vi "Get sr850 Formated Parameters.VI"(8 "error in (no error)":errorcluster, 10 "Initial String":string, 11 "VISA Resource Name":refnum<visa-resource-name>) -> (0 "error out":errorcluster, 1 "Time Constant":dbl format="%.2e", 2 "Sensitivity":dbl format="%.4e", 3 "Frequency":dbl format="%.2e", 4 "Phase":dbl format="%.2f", 5 "Oscillator voltage":dbl format="%.2e", 6 "Parameters":string="SR850 Lockin Settings", 7 "Filter Slope":i32, 9 "Data titles":string[](array[string])=["SRS_Vx (V)", "SRS_Vy (V)"])   [LabVIEW 2015]
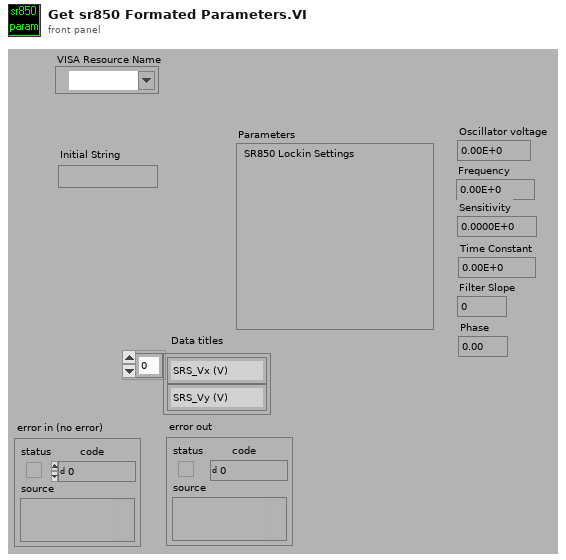
[diagram p1: front panel]
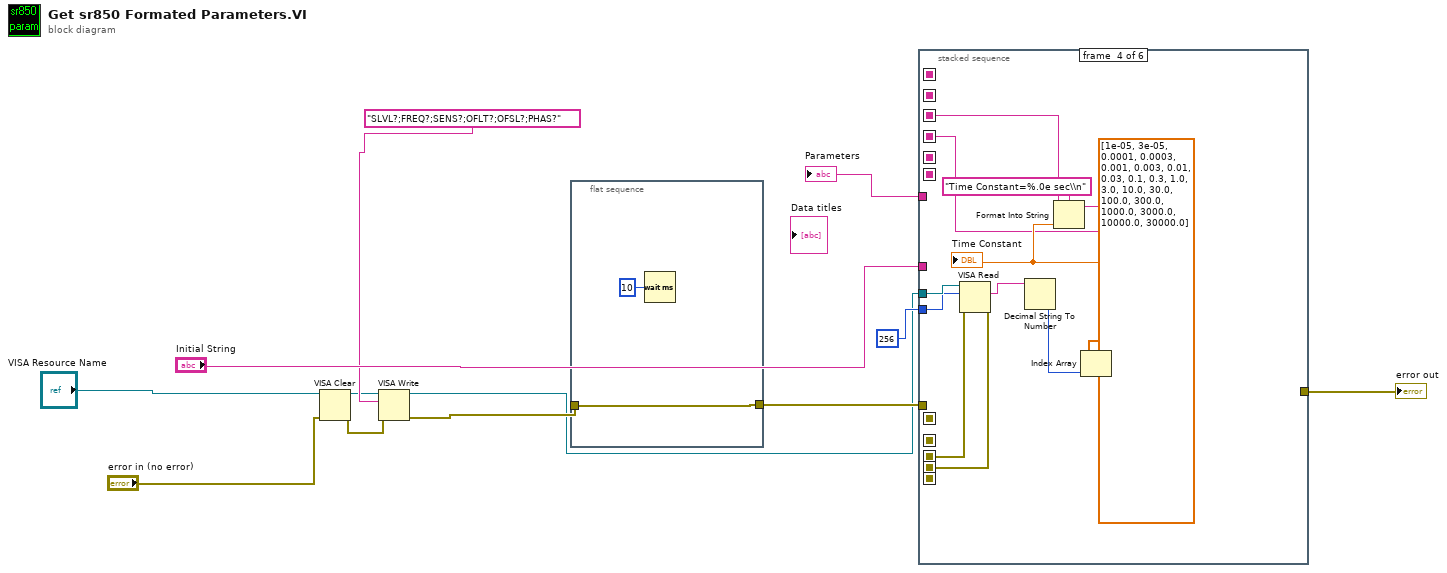
[diagram p0: block diagram]
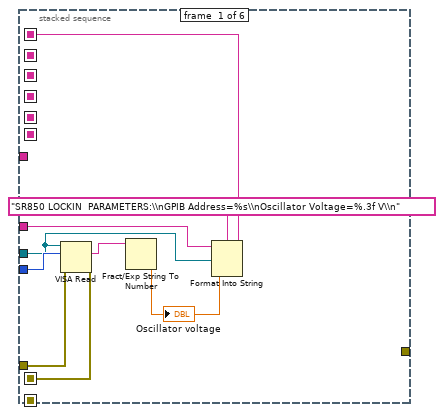
[diagram p2: hidden frame]
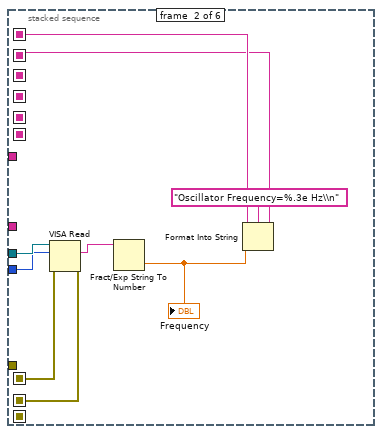
[diagram p3: hidden frame]
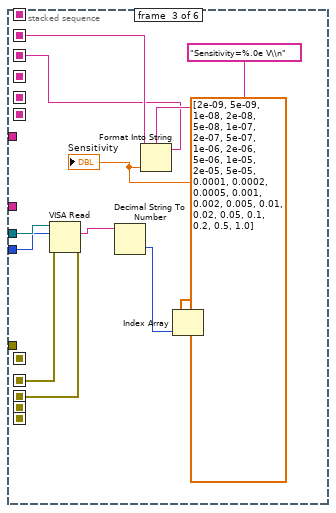
[diagram p4: hidden frame]
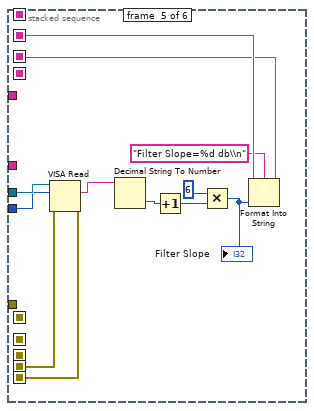
[diagram p5: hidden frame]
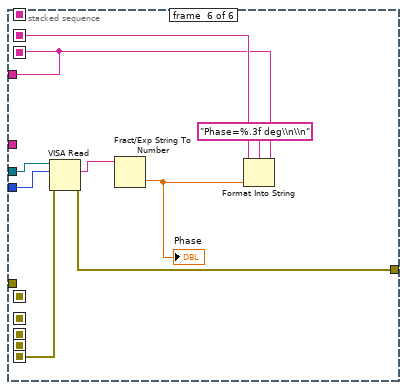
[diagram p6: hidden frame]
diagram:
  n1 = VISA Clear(VISA resource name="VISA Resource Name", error in (no error)="error in (no error)") -> (VISA resource name out=w3:refnum<visa-resource-name>, error out=w6:errorcluster)
  n2 = VISA Write(VISA resource name=w3, write buffer="SLVL?;FREQ?;SENS?;OFLT?;OFSL?;PHAS?" ("data string"), error in (no error)=w6) -> (VISA resource name out=w1:refnum<visa-resource-name>, error out=w5:errorcluster)  [unwired: 1 out]
  n3 = flat-sequence {
    tunnel: [w13] -> w7
    tunnel: w5 -> [w13]
    frame #0 {
      n4 = Wait (ms)(milliseconds to wait=u32 10) -> ()  [unwired: 1 out]
    }
  }
  n5 = stacked-sequence {
    seq-local: [w21 _ _ _ _ _] -> [_ w29 _ _ _ _]
    seq-local: [_ w28 _ _ _ _] -> [_ _ w37 _ _ _]
    seq-local: [_ _ w36 _ _ _] -> [_ _ _ w48 _ _]
    seq-local: [_ _ _ w47 _ _] -> [_ _ _ _ w60 _]
    seq-local: [_ _ _ _ w59 _] -> [_ _ _ _ _ w72]
    seq-local: [_ _ _ _ _ w71] -> [_ _ _ _ _ _]
    seq-local: [w18 _ _ _ _ _] -> [_ w26 _ _ _ _]
    seq-local: [_ w25 _ _ _ _] -> [_ _ w35 _ _ _]
    seq-local: [_ _ w34 _ _ _] -> [_ _ _ w46 _ _]
    seq-local: [_ _ _ w45 _ _] -> [_ _ _ _ w57 _]
    seq-local: [_ _ _ _ w56 _] -> [_ _ _ _ _ w70]
    tunnel: w1 -> [w16 w32 w43 w54 w66 w68]
    tunnel: u32 256 ("count") -> [w23 w27 w42 w53 w65 w75]
    tunnel: [_ _ _ _ _ w71] -> w8
    tunnel: "Initial String" -> [w20 _ _ _ _ _]
    tunnel: w7 -> [w19 _ _ _ _ _]
    tunnel: [_ _ _ _ _ w69] -> w9
    frame #0 {
      n6 = VISA Read(VISA resource name=w16, byte count=w23, error in (no error)=w19) -> (read buffer=w15:string, error out=w18:errorcluster)  [unwired: 2 out]
      n7 = Fract/Exp String To Number(string=w15) -> (number=w17:dbl)  [unwired: 4 out]
      "Oscillator voltage" <- w17
      n8 = Format Into String(format string="SR850 LOCKIN  PARAMETERS:\\nGPIB Address=%s\\nOscillator Voltage=%.3f V\\n", initial string=w20, w16, w17) -> (resulting string=w21:string)  [unwired: 1 in, 1 out]
    }
    frame #1 {
      n9 = VISA Read(VISA resource name=w32, byte count=w27, error in (no error)=w26) -> (read buffer=w24:string, error out=w25:errorcluster)  [unwired: 2 out]
      n10 = Fract/Exp String To Number(string=w24) -> (number=w30:dbl)  [unwired: 4 out]
      "Frequency" <- w30
      n11 = Format Into String(format string="Oscillator Frequency=%.3e Hz\\n", initial string=w29, w30) -> (resulting string=w28:string)  [unwired: 1 in, 1 out]
    }
    frame #2 {
      n12 = VISA Read(VISA resource name=w43, byte count=w42, error in (no error)=w35) -> (read buffer=w33:string, error out=w34:errorcluster)  [unwired: 2 out]
      n13 = Decimal String To Number(string=w33) -> (number=w40:i32)  [unwired: 3 out]
      n14 = Index Array(array=dbl[] [2e-09, 5e-09, 1e-08, 2e-08, 5e-08, 1e-07, 2e-07, 5e-07, 1e-06, 2e-06, 5e-06, 1e-05, 2e-05, 5e-05, 0.0001, 0.0002, 0.0005, 0.001, 0.002, 0.005, 0.01, 0.02, 0.05, 0.1, 0.2, 0.5, 1.0], index=w40) -> (element=w39:dbl)
      "Sensitivity" <- w39
      n15 = Format Into String(format string="Sensitivity=%.0e V\\n", initial string=w37, w39) -> (resulting string=w36:string)  [unwired: 1 in, 1 out]
    }
    frame #3 {
      n16 = VISA Read(VISA resource name=w54, byte count=w53, error in (no error)=w46) -> (read buffer=w44:string, error out=w45:errorcluster)  [unwired: 2 out]
      n17 = Decimal String To Number(string=w44) -> (number=w52:i32)  [unwired: 3 out]
      n18 = Index Array(array=dbl[] [1e-05, 3e-05, 0.0001, 0.0003, 0.001, 0.003, 0.01, 0.03, 0.1, 0.3, 1.0, 3.0, 10.0, 30.0, 100.0, 300.0, 1000.0, 3000.0, 10000.0, 30000.0], index=w52) -> (element=w49:dbl)
      "Time Constant" <- w49
      n19 = Format Into String(format string="Time Constant=%.0e sec\\n", initial string=w48, w49) -> (resulting string=w47:string)  [unwired: 1 in, 1 out]
    }
    frame #4 {
      n20 = VISA Read(VISA resource name=w66, byte count=w65, error in (no error)=w57) -> (read buffer=w55:string, error out=w56:errorcluster)  [unwired: 2 out]
      n21 = Decimal String To Number(string=w55) -> (number=w64:i32)  [unwired: 3 out]
      n22 = Increment(x=w64) -> (x+1=w62:i32)
      n23 = Multiply(x=6, y=w62) -> (x*y=w61:i32)
      "Filter Slope" <- w61
      n24 = Format Into String(format string="Filter Slope=%d db\\n", initial string=w60, w61) -> (resulting string=w59:string)  [unwired: 1 in, 1 out]
    }
    frame #5 {
      n25 = VISA Read(VISA resource name=w68, byte count=w75, error in (no error)=w70) -> (read buffer=w67:string, error out=w69:errorcluster)  [unwired: 2 out]
      n26 = Fract/Exp String To Number(string=w67) -> (number=w74:dbl)  [unwired: 1 in, 3 out]
      "Phase" <- w74
      n27 = Format Into String(format string="Phase=%.3f deg\\n\\n", initial string=w72, w74) -> (resulting string=w71:string)  [unwired: 1 in, 1 out]
    }
  }
  "error out" <- w9
  "Parameters" <- w8
